vi "StopVI.vi"(5 "Signal? [F]":bool, 6 "TimeOut (ms) [-1]":i32=-1, 7 "ForceClose":bool, 8 "error in (no error)":errorcluster, 9 "'Stop' Value":variant, 10 "'Stop' Label":string="Stop", 11 "VI Reference":refnum<vi>) -> (0 "error out":errorcluster, 1 "Timed Out?":bool, 3 "VI Reference (dup)":refnum<vi>)   [LabVIEW 2020]
uses:
  CtlReferences.lvclass/CtlReferences.ctl
  CtlReferences.lvclass
  GetAllControlRefs_Ref.vi
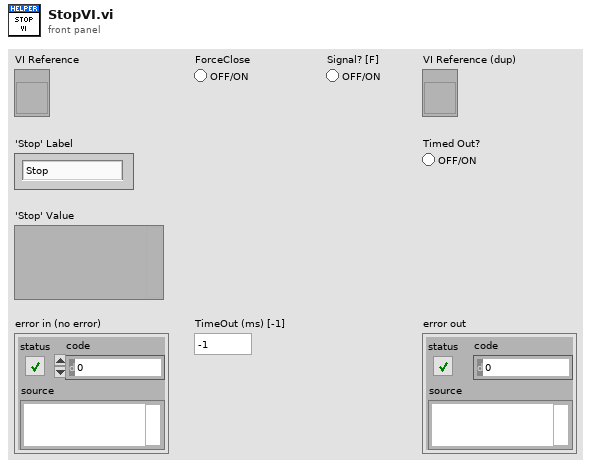
[diagram p1: front panel]
types:
  T1 = enum32{"Bad", "Idle", "Run top level", "Running"}
  T2 = typedef "CtlReferences.lvlib/CtlReferences.lvclass/CtlLookup.ctl" = refnum<data-value>
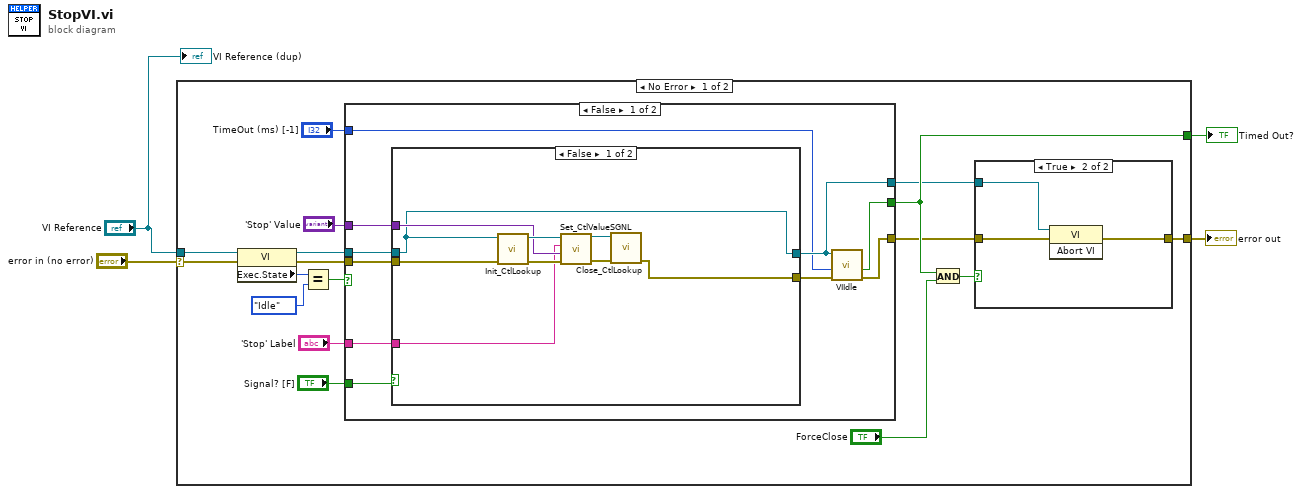
[diagram p0: block diagram]
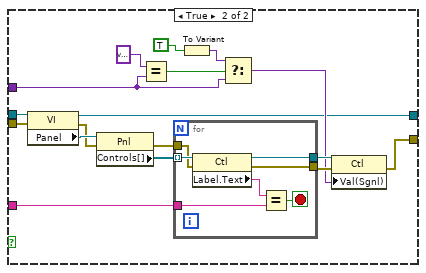
[diagram p3: hidden frame]
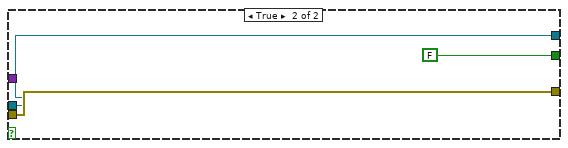
[diagram p4: hidden frame]
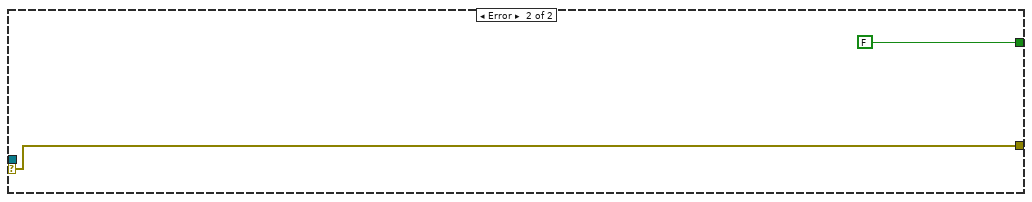
[diagram p5: hidden frame]
diagram:
  n1 = case shown="No Error" "error in (no error)" {
    selector: "error in (no error)" -> [w15 w73]
    tunnel: "VI Reference" -> [w16 _]
    tunnel: [w13 FALSE ("Timed Out?")] -> w3
    tunnel: [w9 w73] -> w2
    frame No Error {
      n2 = property class="VI"(reference=w16, error in=w15) -> (reference out=w17:refnum<vi>, error out=w19:errorcluster, "Exec.State"=w20:T1)
      n3 = Equal?(x=w20, y=T1."Idle" ("Execution:State")) -> (x = y?=w18:bool)
      n4 = case shown="False" w18 {
        tunnel: [w32 w71] -> w11
        tunnel: w19 -> [w35 w71]
        tunnel: w17 -> [w34 w69]
        tunnel: [w31 FALSE ("Timed Out?")] -> w13
        tunnel: [w30 w69] -> w10
        tunnel: "'Stop' Value" -> [w29 _]
        tunnel: "'Stop' Label" -> [w28 _]
        tunnel: "TimeOut (ms) [-1]" -> [w27 _]
        tunnel: "Signal? [F]" -> [w26 _]
        frame False {
          n5 = case shown="False" w26 {
            tunnel: w35 -> [w40 w50]
            tunnel: w34 -> [w36 w49]
            tunnel: [w39 w48] -> w33
            tunnel: [w36 w47] -> w30
            tunnel: w29 -> [w38 w46]
            tunnel: w28 -> [w37 w45]
            frame False {
              n6 = call-poly "Init_CtlLookup.vi"("error in (no error)"=w40, "VI Ref"=w36) -> ("error out"=w42:errorcluster, "CtlLookup Out"=w41:T2)  [unwired: 8 in]
              n7 = call "Set_CtlValueSGNL.vi"("error in (no error)"=w42, "Value"=w38, "Control Label"=w37, "CtlLookup In"=w41) -> ("error out"=w44:errorcluster, "CtlLookup Out"=w43:T2)  [unwired: 6 in]
              n8 = call "Close_CtlLookup.vi"("error in (no error)"=w44, "CtlLookup In"=w43) -> ("error out"=w39:errorcluster)  [unwired: 9 in]
            }
            frame True {
              n9 = property class="VI"(reference=w49, error in=w50) -> (reference out=w47:refnum<vi>, error out=w58:errorcluster, "Panel"=w61:refnum<vi>)
              n10 = property class="Pnl"(reference=w61, error in=w58) -> (error out=w57:errorcluster, "Controls[]"=w60:refnum<vi>[])  [unwired: 1 out]
              n11 = Equal?(x=variant ("Variant"), y=w46) -> (x = y?=w54:bool)
              n12 = for {
                tunnel: w60 -> [w68] mode=indexing
                tunnel: w45 -> [w66]
                tunnel: [w64] -> w59
                tunnel: w57 -> [w63]
                tunnel: [w62] -> w56
                stop <- w65 stop-if-true
                n13 = property class="Ctl"(reference=w68, error in=w63) -> (reference out=w64:refnum<vi>, error out=w62:errorcluster, "Label.Text"=w67:string)
                n14 = Equal?(x=w67, y=w66) -> (x = y?=w65:bool)
              }
              n15 = To Variant(anything=TRUE) -> (Variant=w52:variant)
              n16 = Select(t=w52, s=w54, f=w46) -> (s? t:f=w51:variant)
              n17 = property class="Ctl"(reference=w59, error in=w56, "Val(Sgnl)"=w51) -> (error out=w48:errorcluster)  [unwired: 1 out]
            }
          }
          n18 = call "VIIdle.vi"("error in (no error)"=w33, "TimeOut (ms) [-1]"=w27, "Vi Ref in"=w30) -> ("error out"=w32:errorcluster, "Timed Out?"=w31:bool)  [unwired: 7 in]
        }
        frame True {
        }
      }
      n19 = And(x=w13, y="ForceClose") -> (x .and. y?=w14:bool)
      n20 = case shown="True" w14 {
        tunnel: w11 -> [w22 w25]
        tunnel: w10 -> [_ w24]
        tunnel: [w22 w23] -> w9
        frame False {
        }
        frame True {
          n21 = invoke class="VI" method="Abort VI"(reference=w24, error in=w25) -> (error out=w23:errorcluster)  [unwired: 1 in, 2 out]
        }
      }
    }
    frame Error {
    }
  }
  "error out" <- w2
  "Timed Out?" <- w3
  "VI Reference (dup)" <- "VI Reference"
